vi "Initialize.vi"(8 "Back-Calculation Gain Kb (1)":dbl=1.0, 9 "Anti-Windup Method (Clamping)":T4, 10 "Output Range":T2, 11 "Gains":T1) -> (3 "PID":T3)   [LabVIEW 2015, in "PID.lvlib"]
uses:
  PID.lvlib
  Anti-Windup Method.ctl
  PID.ctl
  Gains.ctl
  Output Range.ctl
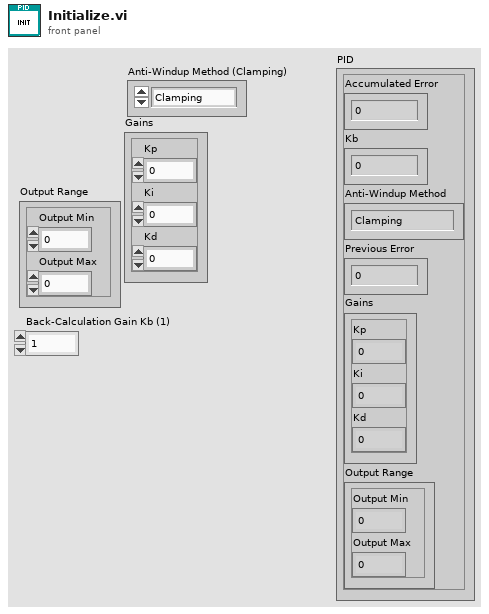
[diagram p1: front panel]
types:
  T1 = typedef "PID.lvlib/Gains.ctl" = cluster{"Kp":dbl, "Ki":dbl, "Kd":dbl}
  T2 = typedef "PID.lvlib/Output Range.ctl" = cluster{"Output Min":dbl, "Output Max":dbl}
  T3 = typedef "PID.lvlib/PID.ctl" = cluster{"Accumulated Error":dbl, "Kb":dbl, "Anti-Windup Method":T4, "Previous Error":dbl, "Gains":T1, "Output Range":T2}
  T4 = typedef "PID.lvlib/Anti-Windup Method.ctl" = enum16{"Clamping", "Back-Calculation", "None"}
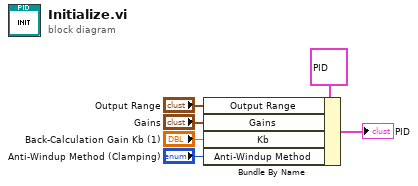
[diagram p0: block diagram]
diagram:
  n1 = Bundle By Name(cluster=T3 {"Accumulated Error"=0.0, "Kb"=0.0, "Anti-Windup Method"=enum."Clamping", "Previous Error"=0.0, "Gains"={"Kp"=0.0, "Ki"=0.0, "Kd"=0.0}, "Output Range"={"Output Min"=0.0, "Output Max"=0.0}} ("PID"), "Output Range"="Output Range", "Gains"="Gains", "Kb"="Back-Calculation Gain Kb (1)", "Anti-Windup Method"="Anti-Windup Method (Clamping)") -> (→"PID":T3)
